vi "Read timing.vi"(8 "error in (no error)":errorcluster, 11 "DSFPlugin in":refnum<class "DSFPlugin.lvclass">) -> (0 "error out":errorcluster, 2 "DSFTiming.lvclass":refnum<class "DSFTiming.lvclass">, 3 "DSFPlugin out":refnum<class "DSFPlugin.lvclass">)   [LabVIEW 2017, in "DSFPlugin.lvclass"]
uses:
  DSFPlugin.lvclass
  DSFTiming/DSFTiming.lvclass
  DSFPlugin.lvclass/DSFPlugin.ctl
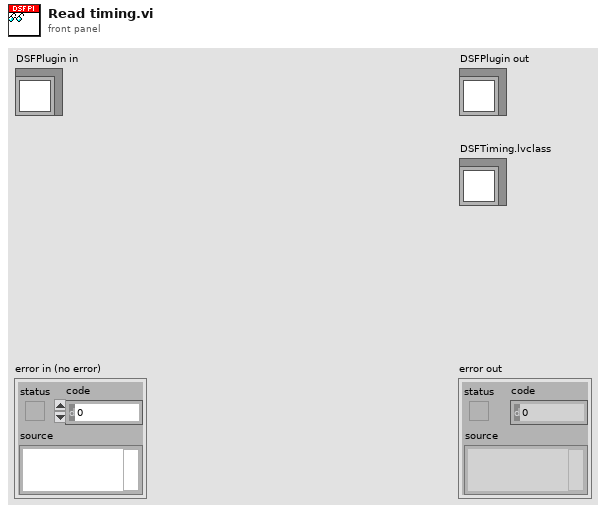
[diagram p1: front panel]
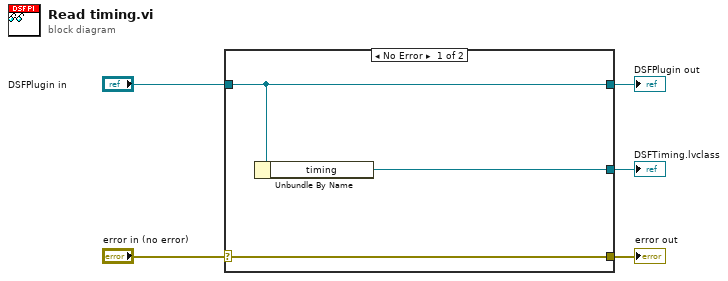
[diagram p0: block diagram]
diagram:
  n1 = case shown="No Error" "error in (no error)" {
    selector: "error in (no error)" -> [w8 w9]
    tunnel: [w8 w9] -> w4
    tunnel: [w7 w10] -> w2
    tunnel: "DSFPlugin in" -> [w7 w10]
    tunnel: [w6 _] -> w1
    frame No Error {
      n2 = Unbundle By Name(w7) -> ("timing"=w6:refnum<class "DSFTiming.lvclass">)
    }
    frame Error {
    }
  }
  "error out" <- w4
  "DSFPlugin out" <- w2
  "DSFTiming.lvclass" <- w1
